vi "Get EST Tunnel and Diagram Ref.vi"(8 "error in (no error)":errorcluster, 10 "FlatSeq Refnum":refnum<vi>, 11 "IO Loop in":refnum<class "Module Loop.lvclass">) -> (0 "error out":errorcluster, 3 "IO Loop out":refnum<class "Module Loop.lvclass">)   [LabVIEW 2015, in "Module Loop.lvclass"]
uses:
  Module Loop.lvclass
  Structures/Structures.lvclass/Structures.ctl
  Structures/Write Structure.vi
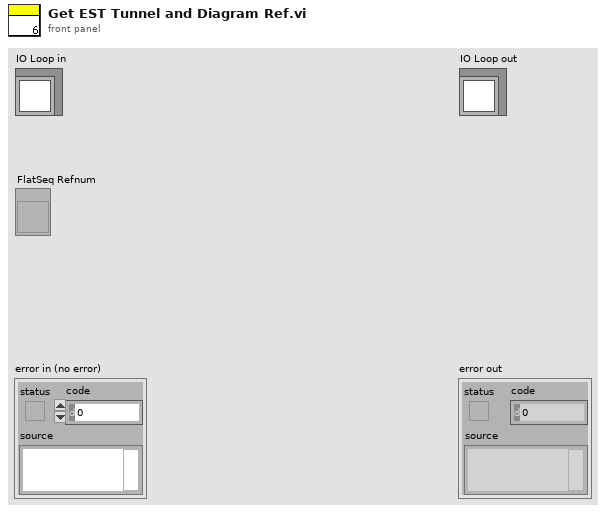
[diagram p1: front panel]
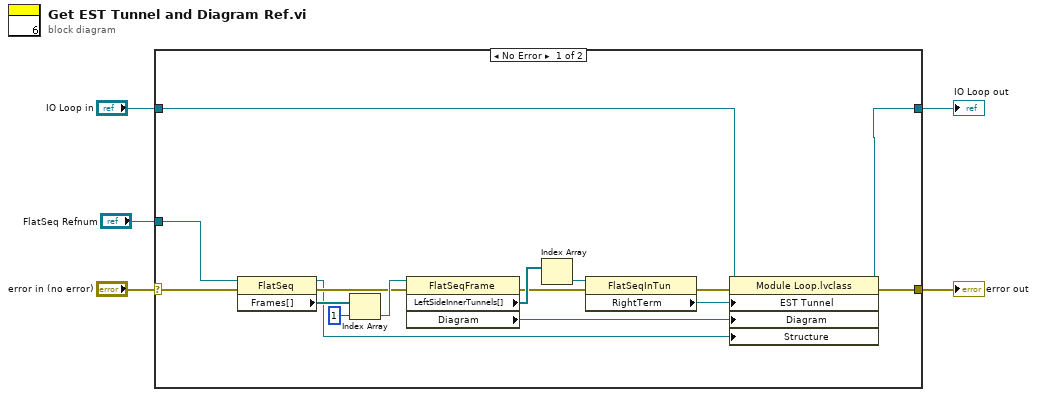
[diagram p0: block diagram]
diagram:
  n1 = case shown="No Error" "error in (no error)" {
    selector: "error in (no error)" -> [w9 w23]
    tunnel: [w8 w23] -> w4
    tunnel: [w10 w22] -> w2
    tunnel: "IO Loop in" -> [w11 w22]
    tunnel: "FlatSeq Refnum" -> [w7 _]
    frame No Error {
      n2 = property class="FlatSeq"(reference=w7, error in=w9) -> (reference out=w6:refnum<vi>, error out=w18:errorcluster, "Frames[]"=w21:refnum<vi>[])
      n3 = Index Array(array=w21, index=1) -> (element=w19:refnum<vi>)
      n4 = property class="FlatSeqFrame"(reference=w19, error in=w18) -> (error out=w15:errorcluster, "LeftSideInnerTunnels[]"=w17:refnum<vi>[], "Diagram"=w14:refnum<vi>)  [unwired: 1 out]
      n5 = Index Array(array=w17) -> (element=w16:refnum<vi>)  [unwired: 1 in]
      n6 = property class="FlatSeqInTun"(reference=w16, error in=w15) -> (error out=w12:errorcluster, "RightTerm"=w13:refnum<vi>)  [unwired: 1 out]
      n7 = property class="Module Loop.lvclass"(reference=w11, error in=w12, "EST Tunnel"=w13, "Diagram"=w14, "Structure"=w6) -> (reference out=w10:refnum<class "Module Loop.lvclass">, error out=w8:errorcluster)
    }
    frame Error {
    }
  }
  "error out" <- w4
  "IO Loop out" <- w2
